vi "BRig_dataExp_BUR_max.vi"() -> (2 "output_BUR_max":i32)   [LabVIEW 2014]
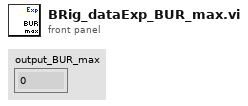
[diagram p1: front panel]
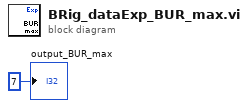
[diagram p0: block diagram]
diagram:
  "output_BUR_max" <- 7 ("output_iBlock")
